vi "Instrument.Framework-Template.Public API.vi"(8 "error in (no error)":errorcluster, 11 "Instrument.Framework-Template in":refnum<class "Instrument.Framework-Template.lvclass">) -> (0 "error out":errorcluster, 2 "commands (this level)":string[](array[string]), 3 "Instrument.Framework-Template out":refnum<class "Instrument.Framework-Template.lvclass">)   [LabVIEW 2019, in "Instrument.Framework-Template.lvclass"]
doc: "Override this VI to return a list of commands only supported by your Instrument"
uses:
  Instrument.Framework-Template.lvclass
  Typedefs/Instrument.Framework-Template.PublicCommands--Enum.ctl
  1e57b0b4-cdd3-4980-bcc7-1b074e876908.vi
  <vilib>/Utility/Data Type/Get Type Information.vi
  <vilib>/Utility/Data Type/Get Numeric Information.vi
  <userlib>/_OpenG.lib/lvdata/lvdata.llb/Unwrap VVariant__ogtk.vi
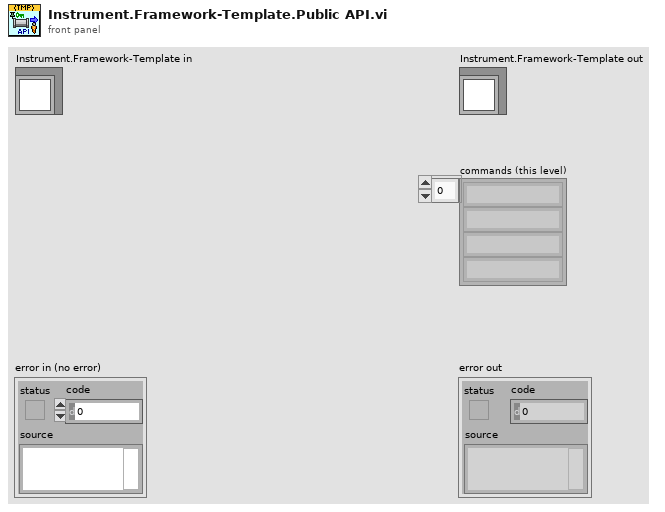
[diagram p1: front panel]
types:
  T1 = typedef "Instrument.Framework-Template.lvclass/Instrument.Framework-Template.PublicCommands--Enum.ctl" = enum16{"doSomething"}
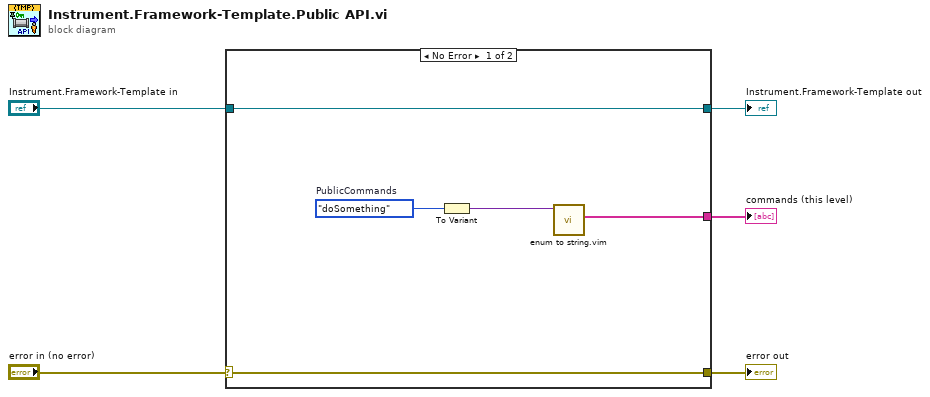
[diagram p0: block diagram]
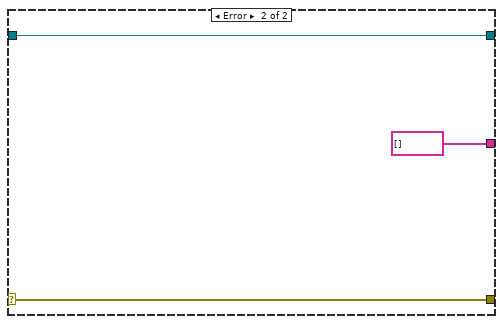
[diagram p2: hidden frame]
diagram:
  n1 = case shown="No Error" "error in (no error)" {
    selector: "error in (no error)" -> [w8 w13]
    tunnel: [w8 w13] -> w4
    tunnel: [w9 w12] -> w1
    tunnel: "Instrument.Framework-Template in" -> [w9 w12]
    tunnel: [w10 string[] [] ("Array")] -> w2
    frame No Error {
      w6 = Instrument.Framework-Template.PublicCommands--Enum."doSomething"  # PublicCommands
      n2 = To Variant(anything=w6) -> (Variant=w7:variant)
      n3 = call "enum to string.vim"("enum in"=w7) -> ("strings out"=w10:string[])  [unwired: 9 in, 1 out]
    }
    frame Error {
    }
  }
  "error out" <- w4
  "Instrument.Framework-Template out" <- w1
  "commands (this level)" <- w2
